vi "UTIL_Login v1_0_0.vi"(8 "error in (no error)":errorcluster, 11 "DB Ref":T1) -> (0 "error out":errorcluster={"status"=TRUE, "code"=8888, "source"="An unsuccessful atempt to login has been made!\nthe user attempted to login as:\rUser: \rPassword: "}, 2 "login":T2={"ProgramPath"=path "", "DataPath"=path "", "DataFileNumber"=-1, "port"="", "User Name"="", "User Level"="", "Login Password"="", "Login Name"="", "Successful?"=FALSE, "Level ID"=""})   [LabVIEW 2009]
doc: "UTIL_Login v1_0_0.vi\n\nThis VI is used as a login security. It is not case sensitive. Type a user name then hit the enter key, then type a password and hit the enter key. If a valid match exits, the VI exits with a true state. If it is invalid the user is prompted with \"Invalid Login\"\n\nTo Modify the user information and passowrd use the database.\n\nCreated By J. Daren Suntych\nNational Analytics 2002\n970-397-0764"
uses:
  <vilib>/addons/database/Connection.llb/Conn ObjectReference.ctl
  <vilib>/addons/database/NI_Database_API.lvlib
panel:
  out "Bad Pass":string
  out "Bad User":string
  in  "Cancel":bool
  in  "Password":string caption="Password:"
  in  "User":string caption="User:"
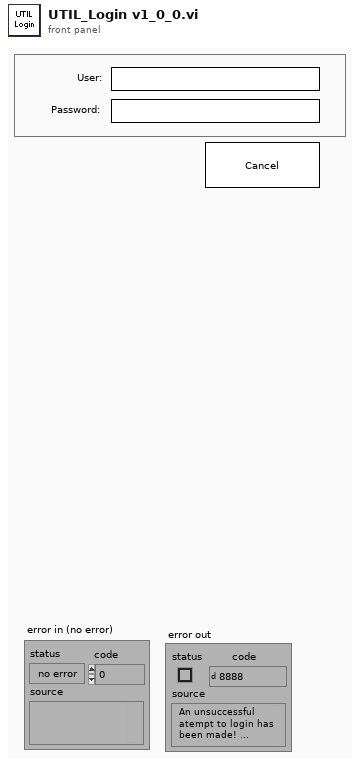
[diagram p1: front panel]
types:
  T1 = typedef "NI_Database_API.lvlib/Conn ObjectReference.ctl" = refnum<k1>
  T2 = cluster{"ProgramPath":path, "DataPath":path, "DataFileNumber":i32, "port":string, "User Name":string, "User Level":string, "Login Password":string, "Login Name":string, "Successful?":bool, "Level ID":string}
  T3 = typedef "Window Refnum" = refnum<k1>
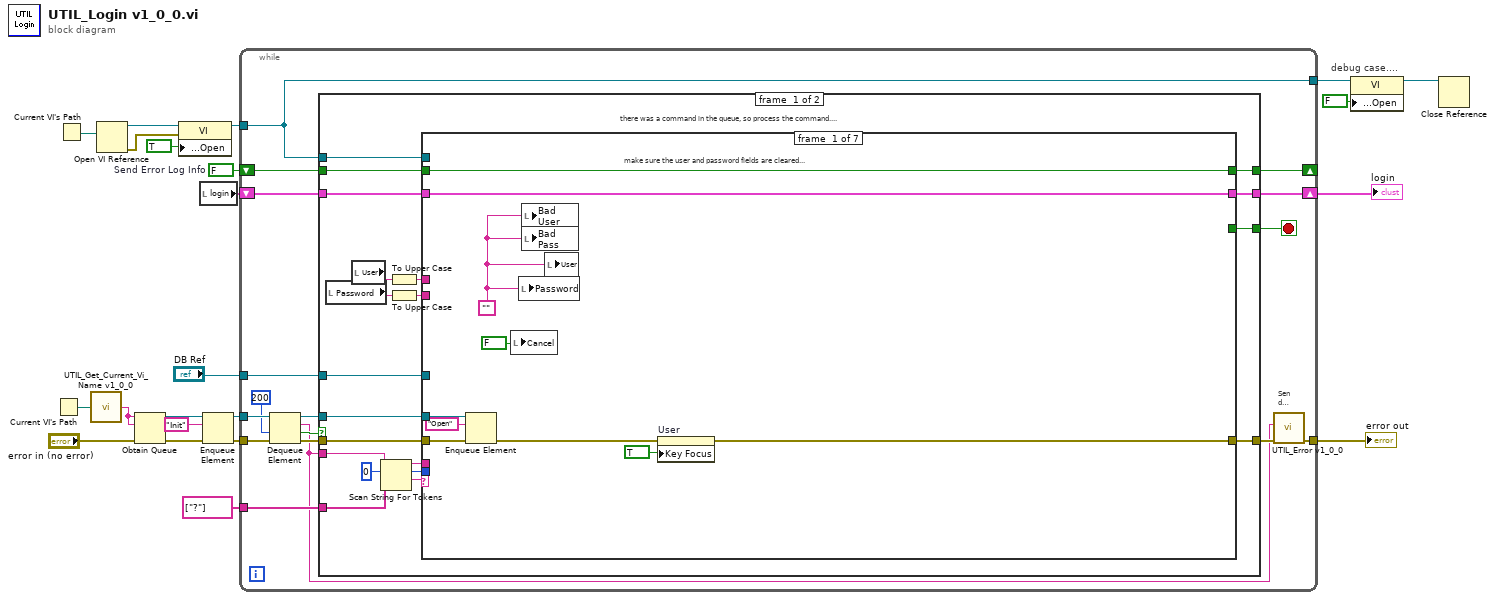
[diagram p0: block diagram]
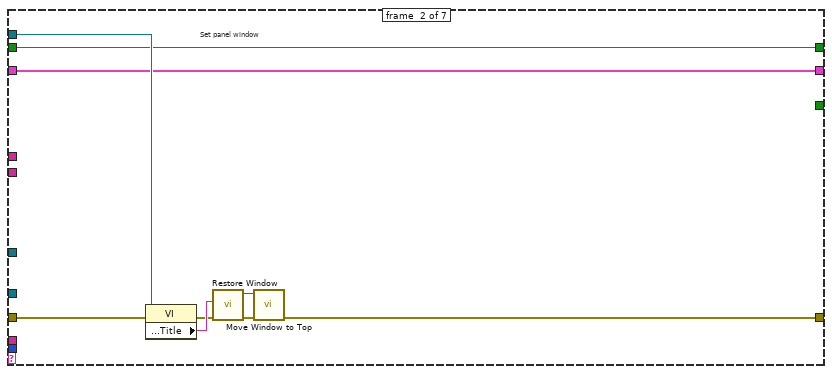
[diagram p2: hidden frame]
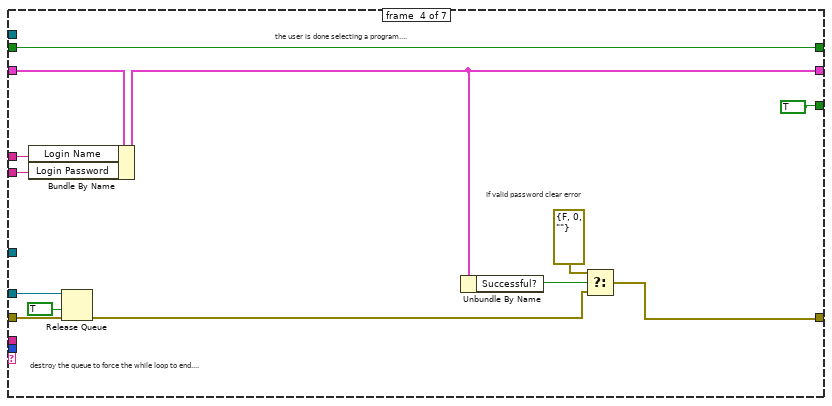
[diagram p4: hidden frame]
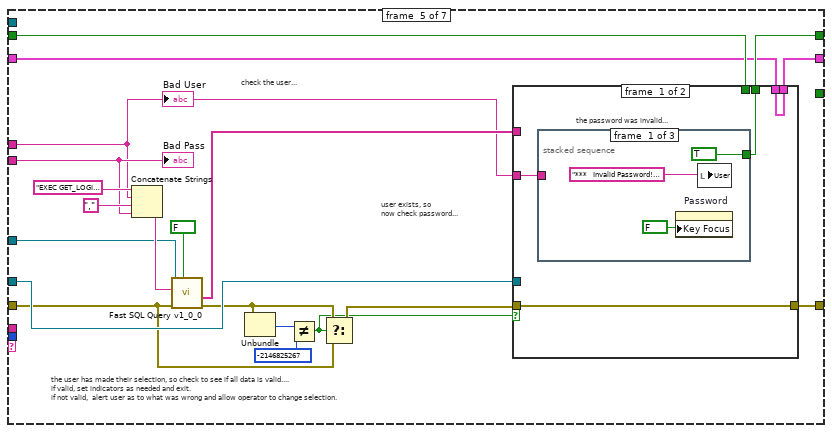
[diagram p5: hidden frame]
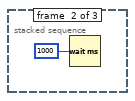
[diagram p6: hidden frame]
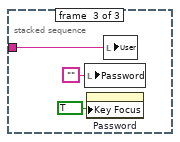
[diagram p7: hidden frame]
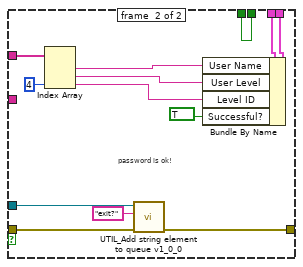
[diagram p8: hidden frame]
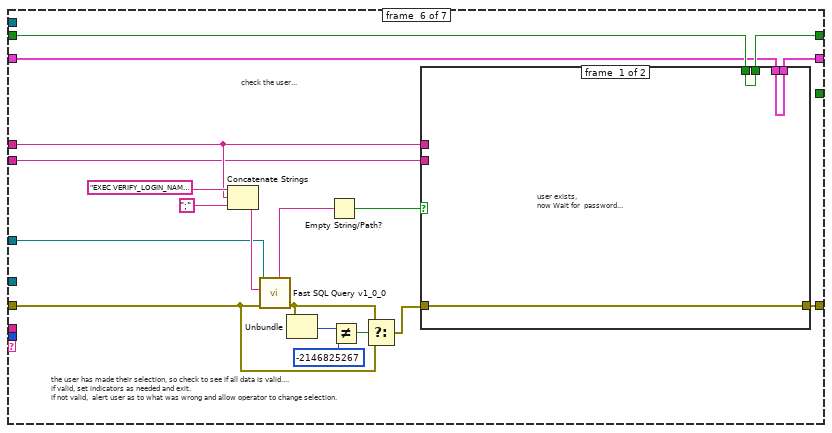
[diagram p9: hidden frame]
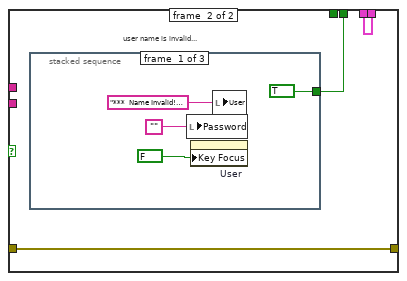
[diagram p10: hidden frame]
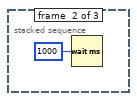
[diagram p11: hidden frame]
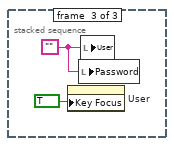
[diagram p12: hidden frame]
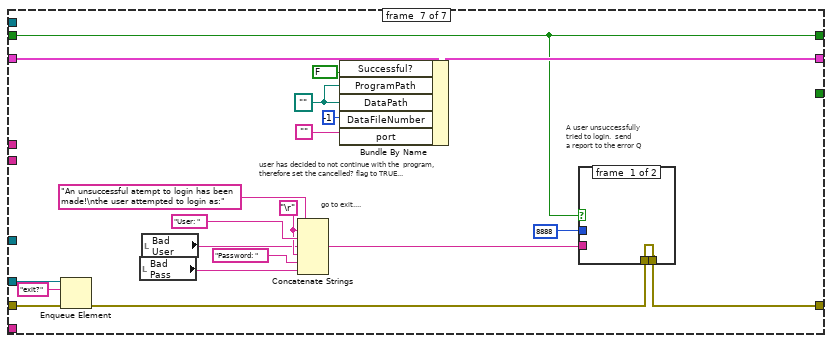
[diagram p13: hidden frame]
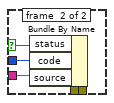
[diagram p14: hidden frame]
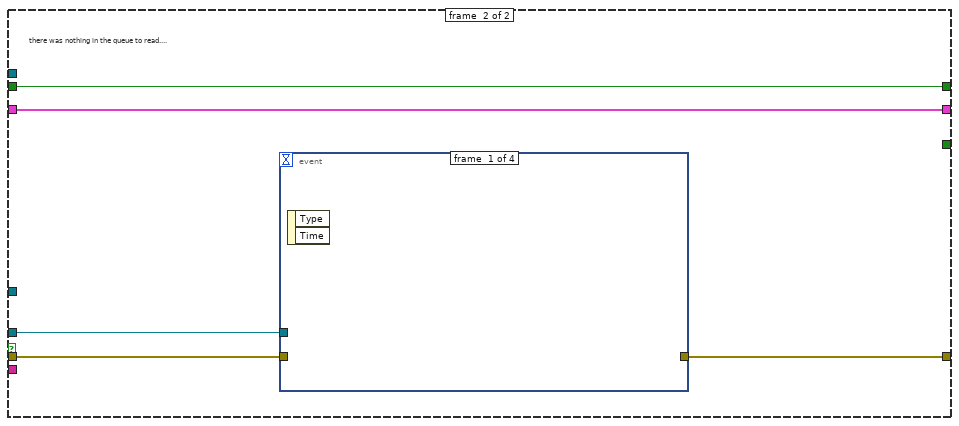
[diagram p15: hidden frame]
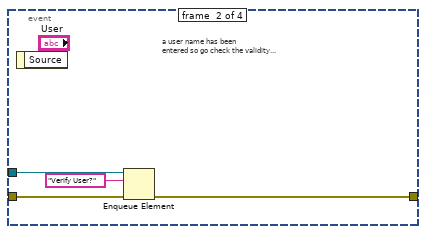
[diagram p16: hidden frame]
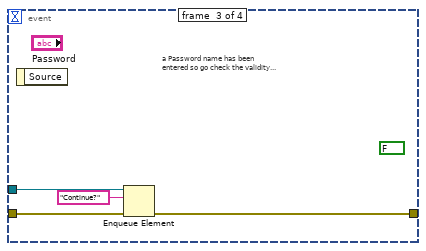
[diagram p17: hidden frame]
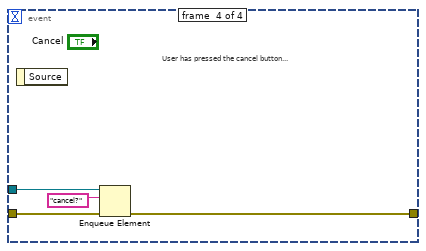
[diagram p18: hidden frame]
diagram:
  w11 = FALSE  # Send Error Log Info
  # "debug case...."
  n1 = Current VI's Path() -> (path=w3:path)
  n2 = Current VI's Path() -> (path=w17:path)
  n3 = call "UTIL_Get_Current_Vi_Name v1_0_0.vi"("Path"=w3) -> ("Name Minus Extention"=w1:string)  [unwired: 2 in, 12 out]
  n4 = Open VI Reference(vi path=w17) -> (vi reference=w15:refnum<vi>, error out=w13:errorcluster)  [unwired: 1 in, 4 out]
  n5 = Obtain Queue(name (unnamed)=w1, element data type=w1, error in (no error)="error in (no error)") -> (queue out=w21:refnum<queue>, error out=w18:errorcluster)  [unwired: 2 in, 1 out]
  n6 = property class="VI"(reference=w15, error in=w13, "Front Panel Window:Open"=TRUE) -> (reference out=w14:refnum<vi>)  [unwired: 1 out]
  n7 = local read "login"() -> (w19:T2)
  n8 = Enqueue Element(queue=w21, element="Init" ("queue element"), error in (no error)=w18) -> (queue out=w10:refnum<queue>, error out=w9:errorcluster)  [unwired: 2 out]
  n9 = while {
    shift-left: w19 -> [w35]
    shift-right: [w34] -> w5
    tunnel: string[] ["?"] ("delimiters (\\s,\\t,\\r,\\n)") -> [w37]
    tunnel: w10 -> [w39]
    tunnel: w14 -> [w33]
    tunnel: [w33] -> w16
    shift-right: [w31] -> _
    shift-left: w11 -> [w32]
    tunnel: w9 -> [w30]
    tunnel: [w26] -> w8
    tunnel: "DB Ref" -> [w23]
    stop <- w28 stop-if-true
    # "Send\nError"
    n10 = Dequeue Element(queue=w39, timeout in ms (-1)=200 ("ms timeout (-1)"), error in (no error)=w30) -> (queue out=w36:refnum<queue>, element=w25:string, timed out?=w38:bool, error out=w29:errorcluster)
    n11 = case shown="False" w38 {
      tunnel: w25 -> [w41 _]
      tunnel: w37 -> [w59 _]
      tunnel: w36 -> [w54 w201]
      tunnel: w35 -> [w53 w199]
      tunnel: [w52 w199] -> w34
      tunnel: [w51 w200] -> w27
      tunnel: w33 -> [w48 _]
      tunnel: w32 -> [w47 w198]
      tunnel: [w46 w198] -> w31
      tunnel: w29 -> [w45 w197]
      tunnel: [w44 _] -> w28
      tunnel: w23 -> [w40 _]
      frame #0 {
        # "there was a command in the queue, so process the command...."
        n12 = local read "Password"() -> (w42:string)
        n13 = local read "User"() -> (w43:string)
        n14 = Scan String For Tokens(6:w59, 8:0 ("offset"), 9:w41) -> (1:w57:string, 2:w56:i32, 3:w55:string)  [unwired: 4 out]
        n15 = To Upper Case(1:w43) -> (0:w50:string)
        n16 = To Upper Case(1:w42) -> (0:w49:string)
        n17 = case shown="Default" w57 {
          tunnel: w56 -> [_ _ _ _ _ _ _]
          tunnel: w55 -> [_ _ _ _ _ _ _]
          tunnel: w50 -> [_ _ _ w86 w96 w151 _]
          tunnel: w49 -> [_ _ _ w84 w97 w150 _]
          tunnel: w54 -> [w63 _ _ w94 w109 _ w185]
          tunnel: w53 -> [w68 w70 w81 w85 w111 w154 w190]
          tunnel: [w68 w70 w81 w82 w110 w153 w189] -> w52
          tunnel: [w65 w71 w79 w93 w112 w155 w183] -> w51
          tunnel: w48 -> [_ w76 _ _ _ _ _]
          tunnel: w47 -> [w69 w75 w80 w90 w113 w156 w182]
          tunnel: [w69 w75 w80 w90 w114 w157 w182] -> w46
          tunnel: w45 -> [w64 w72 w79 w89 w99 w141 w175]
          tunnel: [_ _ _ TRUE ("force destroy? (F)") _ _ _] -> w44
          tunnel: w40 -> [_ _ _ _ w105 w145 _]
          frame #0 {
            w60 = ""
            # "make sure the user and password fields are cleared..."
            n18 = Enqueue Element(queue=w63, element="Open", error in (no error)=w64) -> (error out=w61:errorcluster)  [unwired: 3 out]
            n19 = local write "Cancel"(FALSE ("Continue")) -> ()
            n20 = local write "Password"(w60) -> ()
            n21 = local write "Bad User"(w60) -> ()
            n22 = local write "Bad Pass"(w60) -> ()
            n23 = local write "User"(w60) -> ()
            n24 = property on="User" class="String"(error in=w61, "Key Focus"=TRUE ("Write Attribute")) -> (error out=w65:errorcluster)  [unwired: 1 in, 1 out]
          }
          frame #1 {
            # "Set panel window"
            n25 = property class="VI"(reference=w76, error in=w72) -> (error out=w74:errorcluster, "Front Panel Window:Title"=w77:string)  [unwired: 1 out]
            n26 = call "Restore Window.vi"("error in (no error)"=w74, "window name  (\"\")"=w77) -> ("error out"=w73:errorcluster, "window refnum out"=w78:T3)  [unwired: 1 in, 3 out]
            n27 = call "Move Window to Top.vi"("error in (no error)"=w73, "window refnum (NaWR)"=w78) -> ("error out"=w71:errorcluster)  [unwired: 2 in, 3 out]
          }
          frame #2 {
          }
          frame #3 {
            # "If valid password clear error"
            # "the user is done selecting a program...."
            # "destroy the queue to force the while loop to end...."
            n28 = Bundle By Name(cluster=w85, "Login Name"=w86, "Login Password"=w84) -> (w82:T2)
            n29 = Release Queue(queue=w94, force destroy? (F)=TRUE, error in (no error)=w89) -> (error out=w88:errorcluster)  [unwired: 2 out]
            n30 = Unbundle By Name(w82) -> ("Successful?"=w83:bool)
            n31 = Select(t=errorcluster {"status"=FALSE, "code"=0, "source"=""} ("error out"), s=w83, f=w88) -> (s? t:f=w93:errorcluster)
          }
          frame #4 {
            # "user exists, so\nnow check password..."
            # "the user has made their selection, so check to see if all data is valid....\nif valid, set indicators as needed and exit.\nif not valid,  alert user as to what was wrong and allow operator to change selection."
            # "check the user..."
            n32 = Concatenate Strings("EXEC GET_LOGIN " ("SQL"), w96, "," ("string"), w97) -> (w106:string)
            n33 = call "Fast SQL Query v1_0_0.vi"("Transpose?"=FALSE, "error in (no error)"=w99, "SQL"=w106, "connection reference"=w105) -> ("error out"=w101:errorcluster, "1D Data out"=w104:string[])  [unwired: 6 out]
            n34 = Unbundle(w101) -> ("code"=w103:i32)  [unwired: 2 out]
            n35 = Not Equal?(x=w103, y=-2146825267) -> (x != y?=w98:bool)
            n36 = Select(t=w101, s=w98, f=w99) -> (s? t:f=w100:errorcluster)
            n37 = case shown="True" w98 {
              tunnel: w109 -> [_ w128]
              tunnel: [w118 w138] -> w114
              tunnel: w113 -> [_ w138]
              tunnel: w100 -> [w117 w129]
              tunnel: [w117 w126] -> w112
              tunnel: w111 -> [w116 w137]
              tunnel: [w116 w136] -> w110
              tunnel: w104 -> [_ w135]
              tunnel: w96 -> [w115 _]
              frame #0 {
                # "the password was invalid..."
                n38 = stacked-sequence {
                  tunnel: [TRUE _ _] -> w118
                  tunnel: w115 -> [_ _ w123]
                  frame #0 {
                    n39 = property on="Password" class="String"("Key Focus"=FALSE ("Write Attribute")) -> ()  [unwired: 2 in, 2 out]
                    n40 = local write "User"("***   Invalid Password!  ***" ("Password")) -> ()
                  }
                  frame #1 {
                    n41 = Wait (ms)(milliseconds to wait=u32 1000) -> ()  [unwired: 1 out]
                  }
                  frame #2 {
                    n42 = local write "Password"("") -> ()
                    n43 = property on="Password" class="String"("Key Focus"=TRUE ("Write Attribute")) -> ()  [unwired: 2 in, 2 out]
                    n44 = local write "User"(w123) -> ()
                  }
                }
              }
              frame #1 {
                # "password is ok!"
                n45 = Index Array(array=w135, index #3=4 ("index")) -> (element #1=w134:string, element #2=w133:string, element #3=w130:string)  [unwired: 2 in]
                n46 = call "UTIL_Add string element to queue v1_0_0.vi"("error in (no error)"=w129, "enqueue string"="exit?" ("queue element"), "Queue in"=w128) -> ("error out"=w126:errorcluster)  [unwired: 2 in, 6 out]
                n47 = Bundle By Name(cluster=w137, "User Name"=w134, "User Level"=w133, "Level ID"=w130, "Successful?"=TRUE ("cancelled?")) -> (w136:T2)
              }
            }
            "Bad User" <- w96
            "Bad Pass" <- w97
          }
          frame #5 {
            # "the user has made their selection, so check to see if all data is valid....\nif valid, set indicators as needed and exit.\nif not valid,  alert user as to what was wrong and allow operator to change selection."
            # "check the user..."
            n48 = Concatenate Strings("EXEC VERIFY_LOGIN_NAME " ("SQL"), w151, ";" ("string")) -> (w149:string)
            n49 = call "Fast SQL Query v1_0_0.vi"("error in (no error)"=w141, "SQL"=w149, "connection reference"=w145) -> ("error out"=w140:errorcluster, "Single Out"=w147:string)  [unwired: 1 in, 6 out]
            n50 = Unbundle(w140) -> ("code"=w144:i32)  [unwired: 2 out]
            n51 = Empty String/Path?(string/path=w147) -> (empty?=w146:bool)
            n52 = Not Equal?(x=w144, y=-2146825267) -> (x != y?=w142:bool)
            n53 = Select(t=w140, s=w142, f=w141) -> (s? t:f=w139:errorcluster)
            n54 = case shown="True" w146 {
              tunnel: w150 -> [_ _]
              tunnel: w151 -> [_ _]
              tunnel: [w158 w163] -> w157
              tunnel: w156 -> [w158 _]
              tunnel: w139 -> [w160 w162]
              tunnel: [w160 w162] -> w155
              tunnel: w154 -> [w159 w161]
              tunnel: [w159 w161] -> w153
              frame #0 {
                # "user exists, \nnow Wait for  password..."
              }
              frame #1 {
                # "user name is invalid..."
                n55 = stacked-sequence {
                  tunnel: [TRUE _ _] -> w163
                  frame #0 {
                    n56 = local write "Password"("") -> ()
                    n57 = property on="User" class="String"("Key Focus"=FALSE ("Write Attribute")) -> ()  [unwired: 2 in, 2 out]
                    n58 = local write "User"("***  Name Invalid!  ***" ("User")) -> ()
                  }
                  frame #1 {
                    n59 = Wait (ms)(milliseconds to wait=u32 1000) -> ()  [unwired: 1 out]
                  }
                  frame #2 {
                    w170 = ""
                    n60 = property on="User" class="String"("Key Focus"=TRUE ("Write Attribute")) -> ()  [unwired: 2 in, 2 out]
                    n61 = local write "Password"(w170) -> ()
                    n62 = local write "User"(w170) -> ()
                  }
                }
              }
            }
          }
          frame #6 {
            w178 = "\r"
            w188 = path "" ("program")
            # "A user unsuccessfully\ntried to login.  send\na report to the error Q"
            # "go to exit...."
            # "user has decided to not continue with the  program,\ntherefore set the cancelled? flag to TRUE..."
            n63 = Enqueue Element(queue=w185, element="exit?" ("queue element"), error in (no error)=w175) -> (error out=w174:errorcluster)  [unwired: 3 out]
            n64 = local read "Bad Pass"() -> (w171:string)
            n65 = local read "Bad User"() -> (w172:string)
            n66 = Concatenate Strings("An unsuccessful atempt to login has been made!\nthe user attempted to login as:" ("source"), w178, "User: " ("source"), w172, w178, "Password: " ("source"), w171) -> (w176:string)
            n67 = Bundle By Name(cluster=w190, "Successful?"=FALSE ("cancelled?"), "ProgramPath"=w188, "DataPath"=w188, "DataFileNumber"=-1 ("Bundle Element"), "port"="") -> (w189:T2)
            n68 = case shown="True" w182 {
              selector: w182 -> [_ w194]
              tunnel: w174 -> [w191 w196]
              tunnel: [w191 w195] -> w183
              tunnel: 8888 ("code") -> [_ w193]
              tunnel: w176 -> [_ w192]
              frame #0 {
              }
              frame #1 {
                n69 = Bundle By Name(cluster=w196, "status"=w194, "code"=w193, "source"=w192) -> (w195:errorcluster)
              }
            }
          }
        }
      }
      frame #1 {
        # "there was nothing in the queue to read...."
        n70 = event shown="[2] \"Password\": Value Change" {
          selector: _ -> [_ _ _ _]
          dyn-events: _ -> [_ _ _ _]
          timeout: _ -> [_ _ _ _]
          tunnel: w201 -> [_ w203 w207 w212]
          tunnel: w197 -> [_ w204 w208 w213]
          tunnel: [_ w202 w206 w211] -> w200
          event #0 {
            n71 = event-data() -> ()  [unwired: 3 out]
          }
          event #1 {
            # "a user name has been\nentered so go check the validity..."
            n72 = event-data() -> ()  [unwired: 2 out]
            n73 = Enqueue Element(queue=w203, element="Verify User?" ("queue element"), error in (no error)=w204) -> (error out=w202:errorcluster)  [unwired: 3 out]
          }
          event #2 {
            (unwired) FALSE ("Write Attribute")
            # "a Password name has been\nentered so go check the validity..."
            n74 = event-data() -> ()  [unwired: 2 out]
            n75 = Enqueue Element(queue=w207, element="Continue?" ("queue element"), error in (no error)=w208) -> (error out=w206:errorcluster)  [unwired: 3 out]
          }
          event #3 {
            # "User has pressed the cancel button..."
            n76 = event-data() -> ()  [unwired: 2 out]
            n77 = Enqueue Element(queue=w212, element="cancel?" ("queue element"), error in (no error)=w213) -> (error out=w211:errorcluster)  [unwired: 3 out]
          }
        }
      }
    }
    n78 = call "UTIL_Error v1_0_0.vi"("error in (no error)"=w27, "State"=w25) -> ("error out"=w26:errorcluster)  [unwired: 1 in, 8 out]
  }
  "login" <- w5
  "error out" <- w8
  n79 = property class="VI"(reference=w16, "Front Panel Window:Open"=FALSE) -> (reference out=w7:refnum<vi>)  [unwired: 1 in, 1 out]
  n80 = Close Reference(reference=w7) -> ()  [unwired: 1 in, 1 out]
